vi "Get Steering Motor Angle Setpoint.vi"(8 "error in (no error)":errorcluster, 11 "wheel in":refnum<class "NI_Robotics_Steering Wheel.lvclass">) -> (0 "error out":errorcluster, 1 "failed?":bool, 2 "ccw motor angle setpoint (rad)":dbl, 3 "wheel out":refnum<class "NI_Robotics_Steering Wheel.lvclass">)   [LabVIEW 2017, in "NI_Robotics_Steering Wheel.lvclass"]
uses:
  <vilib>/robotics/Steering/Steering Wheel/NI_Robotics_Steering Wheel.lvclass
  <vilib>/robotics/Steering/Steering Wheel/NI_Robotics_Steering Wheel.lvclass/NI_Robotics_Steering Wheel.ctl
  <vilib>/robotics/Actuation/Motor Communication/NI_Robotics_Motor Communication.lvclass
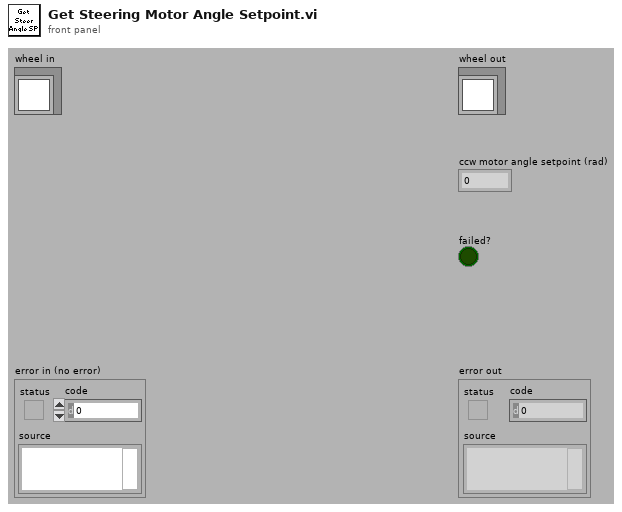
[diagram p1: front panel]
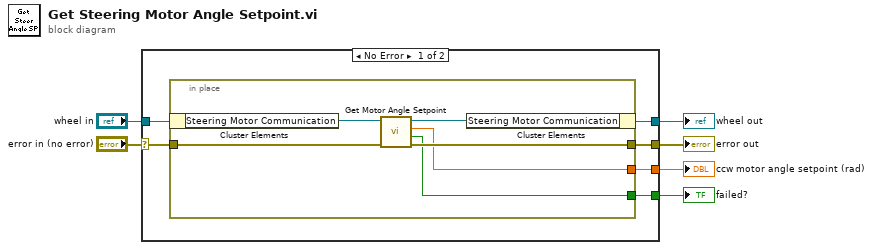
[diagram p0: block diagram]
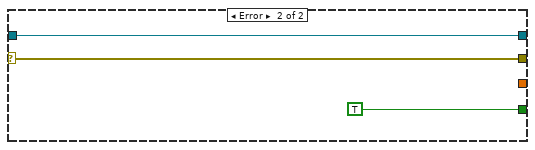
[diagram p2: hidden frame]
diagram:
  n1 = case shown="No Error" "error in (no error)" {
    selector: "error in (no error)" -> [w10 w21]
    tunnel: [w9 w21] -> w3
    tunnel: [w11 w20] -> w5
    tunnel: "wheel in" -> [w12 w20]
    tunnel: [w8 _] -> w1
    tunnel: [w7 TRUE ("failed?")] -> w2
    frame No Error {
      n2 = in-place {
        in-place-border: [w15] -> w9
        in-place-border: w10 -> [w16]
        in-place-border: [w14] -> w8
        in-place-border: [w13] -> w7
        n3 = in-place-cluster #1(w12) -> ("Steering Motor Communication"=w18:refnum<class "NI_Robotics_Motor Communication.lvclass">)
        n4 = call <vilib>:"Get Motor Angle Setpoint.vi"("error in (no error)"=w16, "motor communication in"=w18) -> ("error out"=w15:errorcluster, "failed?"=w13:bool, "angle"=w14:dbl, "motor communication out"=w17:refnum<class "NI_Robotics_Motor Communication.lvclass">)  [unwired: 6 in]
        n5 = in-place-cluster #1("Steering Motor Communication"=w17) -> (w11:refnum<class "NI_Robotics_Steering Wheel.lvclass">)
      }
    }
    frame Error {
    }
  }
  "error out" <- w3
  "wheel out" <- w5
  "ccw motor angle setpoint (rad)" <- w1
  "failed?" <- w2
